vi "Teleop.vi"(10 "Match Info":T1={"Autonomous Elapsed Seconds"=0.0, "TeleOp Elapsed Seconds"=0.0, "Disabled Elapsed Seconds"=0.0, "Visited Autonomous"=FALSE, "Visited TeleOp"=FALSE, "Visited Disabled"=FALSE, "Autonomous Settings"={"Autonomous Style"=enum."Independent", "VI Refnum"=refnum}}, 11 "Call Context":T2) -> ()   [LabVIEW 2013]
doc: "This VI is called for each TeleOp packet received from the DS where the robot is not disabled. It is often used to read from the joysticks and update I/O or to update setpoints for timed control loops. It should complete and return within 20 milliseconds or it may miss DS packets."
uses:
  <vilib>/Rock Robotics/WPI/DriverStation/WPI_DriverStationDerivedRobotMode.ctl
  <vilib>/Rock Robotics/WPI/DriverStation/WPI_DriverStationMatch Info.ctl
  <vilib>/Rock Robotics/WPI/Solenoid/WPI_SolenoidValue.ctl
  Robot Global Data.vi
  <vilib>/Rock Robotics/WPI/Solenoid/Deprecated/WPI_SolenoidGetBool.vi
  <vilib>/Rock Robotics/WPI/Solenoid/WPI_SolenoidSetEnum.vi
  POT.vi
  Voltage.vi
  <vilib>/Rock Robotics/WPI/Joystick/WPI_JoystickGetSetRefNum.vi
  <vilib>/Rock Robotics/WPI/RobotDrive/WPI_RobotDriveGetSetRefNum.vi
panel:
  out "Voltage":dbl
  out "POT Value":dbl
  out "Numeric 1":dbl(slide) scale=0.0..100.0
  out "Boolean 2":bool
  out "Boolean 1":bool
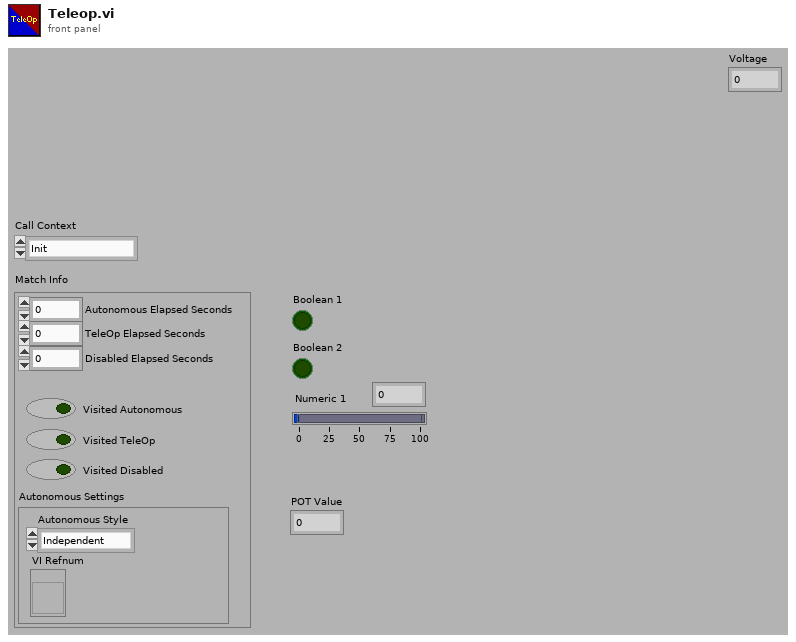
[diagram p1: front panel]
types:
  T1 = typedef "WPI_DriverStationMatch Info.ctl" = cluster{"Autonomous Elapsed Seconds":dbl, "TeleOp Elapsed Seconds":dbl, "Disabled Elapsed Seconds":dbl, "Visited Autonomous":bool, "Visited TeleOp":bool, "Visited Disabled":bool, "Autonomous Settings":cluster{"Autonomous Style":enum16{"Iterative", "Independent"}, "VI Refnum":refnum<vi>}}
  T2 = typedef "WPI_DriverStationDerivedRobotMode.ctl" = enum16{"Init", "Execute", "Stop"}
  T3 = typedef "WPI_JoystickDevRef.ctl" = cluster{"Device":T4}
  T4 = typedef "WPI_JoystickDeviceEnum.ctl" = enum16{"USB 1", "USB 2", "USB 3", "USB 4", "Kinect 1", "Kinect 2"}
  T5 = typedef "WPI_JoystickButtonState.ctl" = cluster{"Button 1":bool, "Button 2":bool, "Button 3":bool, "Button 4":bool, "Button 5":bool, "Button 6":bool, "Button 7":bool, "Button 8":bool, "Button 9":bool, "Button 10":bool, "Button 11":bool, "Button 12":bool}
  T6 = typedef "WPI_RobotDriveDevRef.ctl" = cluster{"DevStatus":errorcluster, "Motors[]":T7[], "Square Inputs":bool, "Max Output":dbl, "Isochronous":bool}
  T7 = typedef "WPI_MotorControlDeviceRef.ctl" = cluster{"DeviceStatus":errorcluster, "Type":enum16{"PWM", "CAN"}, "PWM":cluster{"Digital Module":T8, "PWM Channel":T9, "DeadBand":T10}, "CAN":cluster{"Device Number":u8, "Control Mode":T11, "Semaphore":T12, "Max Vout":dbl}, "Invert":bool, "TransformRef":T13, "InvTransformRef":T13}
  T8 = typedef "FPGA_TypedefDigitalModule.ctl" = enum16{"Digital Module 1", "Digital Module 2"}
  T9 = typedef "FPGA_DIOPWMChannel.ctl" = enum8{"PWM 1", "PWM 2", "PWM 3", "PWM 4", "PWM 5", "PWM 6", "PWM 7", "PWM 8", "PWM 9", "PWM 10", "Invalid"}
  T10 = typedef "WPI_PWMDeadband.ctl" = cluster{"Name":string, "maxPositivePwm":i32, "minPositivePwm":i32, "centerPwm":i32, "maxNegativePwm":i32, "minNegativePwm":i32, "angularRange":u16}
  T11 = typedef "WPI_CANJaguar_ControlMode.ctl" = enum8{"Percent VBus", "Current", "Speed", "Position", "Voltage"}
  T12 = typedef "Semaphore RefNum" = refnum<k1>
  T13 = typedef "WPI_PWMTransform_ConPane.ctl" = refnum<vi>
  T14 = cluster{"axis 1 (x)":dbl, "axis 2 (y)":dbl, "axis 3 (throttle)":dbl, "axis 4":dbl, "axis 5":dbl, "axis 6":dbl}
  T15 = typedef "WPI_SolenoidDevRef.ctl" = cluster{"DevStatus":errorcluster, "Solenoid Module":T16, "Forward Solenoid Channel":T17, "Reverse Solenoid Channel":T17}
  T16 = typedef "FPGA_TypedefSolenoidModule.ctl" = enum16{"Solenoid Module 1", "Solenoid Module 2"}
  T17 = typedef "WPI_SolenoidChannel.ctl" = enum8{"Solenoid 1", "Solenoid 2", "Solenoid 3", "Solenoid 4", "Solenoid 5", "Solenoid 6", "Solenoid 7", "Solenoid 8", "Invalid"}
  T18 = typedef "WPI_SolenoidValue.ctl" = enum16{"Off", "On", "Forward", "Reverse"}
  T19 = typedef "WPI_RelayDevRef.ctl" = cluster{"DevStatus":errorcluster, "Relay Channel":T20, "Digital Module":T8, "Relay Direction":T21}
  T20 = typedef "FPGA_DIORelayChannel.ctl" = enum8{"Relay 1", "Relay 2", "Relay 3", "Relay 4", "Relay 5", "Relay 6", "Relay 7", "Relay 8", "Invalid"}
  T21 = typedef "WPI_RelayDirection.ctl" = enum16{"Both directions", "Forward only", "Reverse only"}
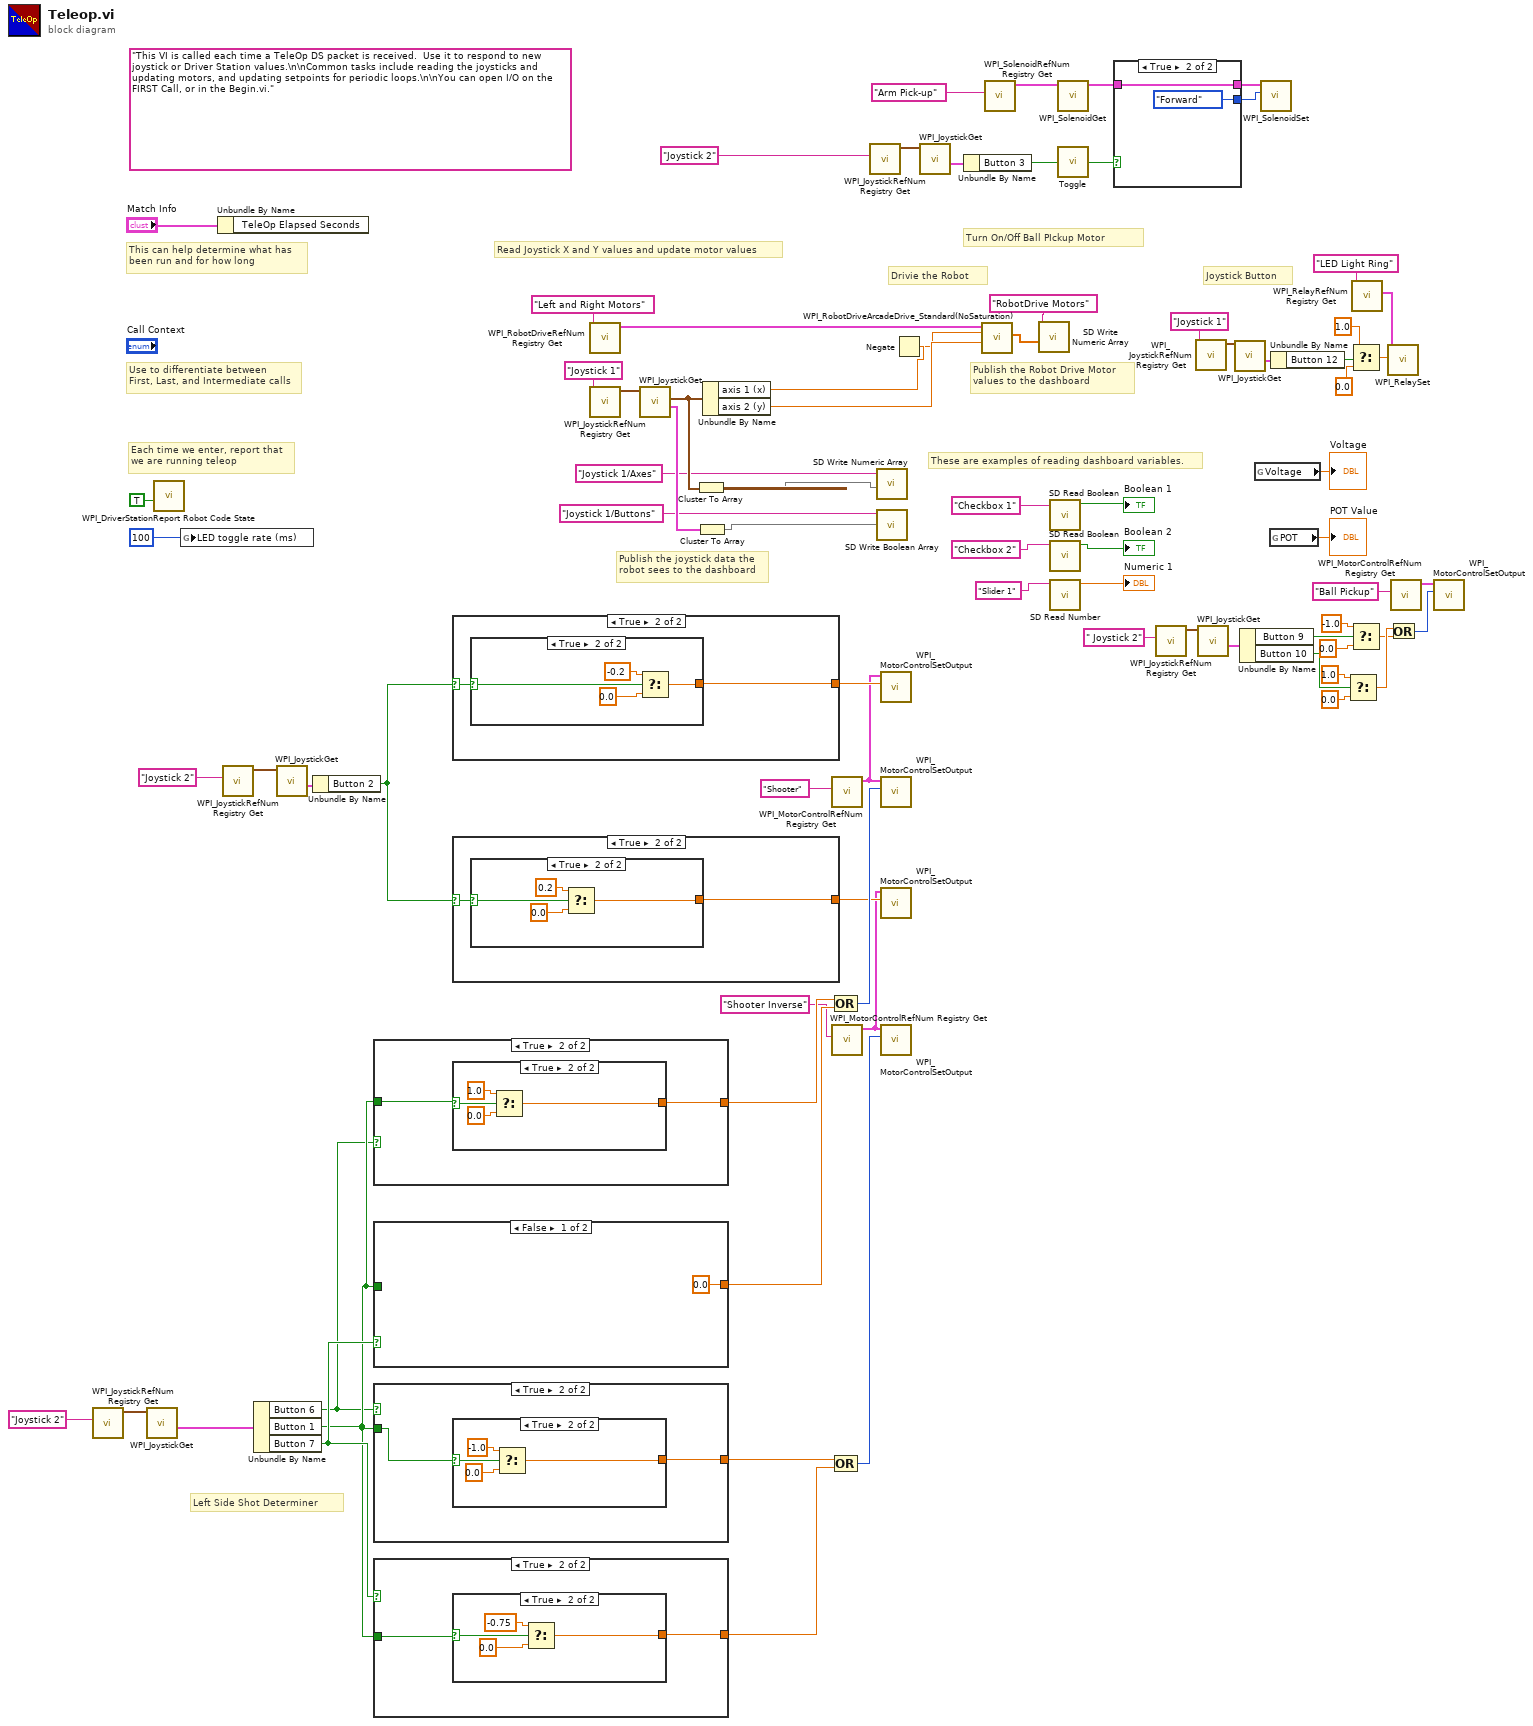
[diagram p0: block diagram]
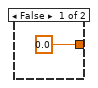
[diagram p2: hidden frame]
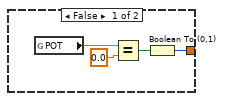
[diagram p3: hidden frame]
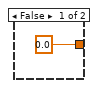
[diagram p4: hidden frame]
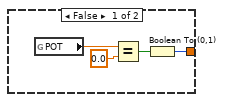
[diagram p5: hidden frame]
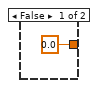
[diagram p6: hidden frame]
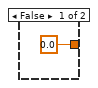
[diagram p7: hidden frame]
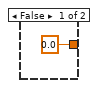
[diagram p8: hidden frame]
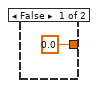
[diagram p9: hidden frame]
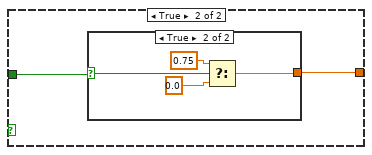
[diagram p10: hidden frame]
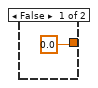
[diagram p11: hidden frame]
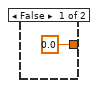
[diagram p12: hidden frame]
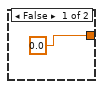
[diagram p13: hidden frame]
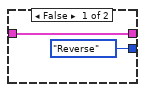
[diagram p14: hidden frame]
diagram:
  (unwired) "This VI is called each time a TeleOp DS packet is received.  Use it to respond to new joystick or Driver Station values.\n\nCommon tasks include reading the joysticks and updating motors, and updating setpoints for periodic loops.\n\nYou can open I/O on the FIRST Call, or in the Begin.vi."
  # "Left Side Shot Determiner"
  # "Turn On/Off Ball PIckup Motor"
  # "Joystick Button"
  # "Drivie the Robot"
  # "These are examples of reading dashboard variables."
  # "Publish the Robot Drive Motor\nvalues to the dashboard"
  # "Publish the joystick data the\nrobot sees to the dashboard"
  # "Each time we enter, report that\nwe are running teleop"
  # "Use to differentiate between\nFirst, Last, and Intermediate calls"
  # "This can help determine what has\nbeen run and for how long"
  # "Read Joystick X and Y values and update motor values"
  n1 = call <vilib>:"WPI_JoystickRefNum Registry Get.vi"("refnum name"="Joystick 2") -> ("JoystickDevRef"=w15:T3)  [unwired: 9 in, 1 out]
  n2 = call <vilib>:"WPI_JoystickGet.vi"("JoystickDevRef"=w15) -> ("Buttons"=w16:T5)  [unwired: 4 in, 2 out]
  n3 = call <vilib>:"WPI_DriverStationReport Robot Code State.vi"("TeleOp"=TRUE ("Autonomous")) -> ()  [unwired: 10 in, 1 out]
  n4 = global write "Robot Global Data.vi" "LED toggle rate (ms)"(u32 100 ("LED ms toggle rate")) -> ()
  n5 = Unbundle By Name("Match Info") -> ()  [unwired: 1 out]
  n6 = call <vilib>:"WPI_JoystickRefNum Registry Get.vi"("refnum name"="Joystick 2") -> ("JoystickDevRef"=w7:T3)  [unwired: 9 in, 1 out]
  n7 = Unbundle By Name(w16) -> ("Button 6"=w1:bool, "Button 1"=w2:bool, "Button 7"=w3:bool)
  n8 = call <vilib>:"WPI_JoystickGet.vi"("JoystickDevRef"=w7) -> ("Buttons"=w5:T5)  [unwired: 4 in, 2 out]
  n9 = Unbundle By Name(w5) -> ("Button 2"=w4:bool)
  n10 = case shown="True" w1 {
    tunnel: [0.0 ("f") w84] -> w20
    tunnel: w2 -> [_ w83]
    frame False {
    }
    frame True {
      n11 = case shown="True" w83 {
        selector: w83 -> [_ w87]
        tunnel: [0.0 ("y") w86] -> w84
        frame False {
        }
        frame True {
          n12 = Select(t=1.0, s=w87, f=0.0) -> (s? t:f=w86:dbl)
        }
      }
    }
  }
  n13 = case shown="False" w3 {
    tunnel: [0.0 ("f") w92] -> w21
    tunnel: w2 -> [_ w91]
    frame False {
    }
    frame True {
      n14 = case shown="True" w91 {
        selector: w91 -> [_ w95]
        tunnel: [0.0 ("y") w94] -> w92
        frame False {
        }
        frame True {
          n15 = Select(t=0.75, s=w95, f=0.0) -> (s? t:f=w94:dbl)
        }
      }
    }
  }
  n16 = case shown="True" w1 {
    tunnel: [0.0 ("f") w100] -> w17
    tunnel: w2 -> [_ w99]
    frame False {
    }
    frame True {
      n17 = case shown="True" w99 {
        selector: w99 -> [_ w103]
        tunnel: [0.0 ("y") w102] -> w100
        frame False {
        }
        frame True {
          n18 = Select(t=-1.0, s=w103, f=0.0) -> (s? t:f=w102:dbl)
        }
      }
    }
  }
  n19 = case shown="True" w3 {
    tunnel: [0.0 ("f") w108] -> w18
    tunnel: w2 -> [_ w107]
    frame False {
    }
    frame True {
      n20 = case shown="True" w107 {
        selector: w107 -> [_ w111]
        tunnel: [0.0 ("y") w110] -> w108
        frame False {
        }
        frame True {
          n21 = Select(t=-0.75, s=w111, f=0.0) -> (s? t:f=w110:dbl)
        }
      }
    }
  }
  n22 = case shown="True" w4 {
    selector: w4 -> [_ w115]
    tunnel: [0.0 ("f") w116] -> w10
    frame False {
    }
    frame True {
      n23 = case shown="True" w115 {
        selector: w115 -> [_ w122]
        tunnel: [w117 w121] -> w116
        frame False {
          n24 = global read "POT.vi" "POT"() -> (w119:dbl)
          n25 = Equal?(x=w119, y=0.0) -> (x = y?=w118:bool)
          n26 = Boolean To (0,1)(Boolean=w118) -> (0, 1=w117:i16)
        }
        frame True {
          n27 = Select(t=-0.2, s=w122, f=0.0) -> (s? t:f=w121:dbl)
        }
      }
    }
  }
  n28 = case shown="True" w4 {
    selector: w4 -> [_ w126]
    tunnel: [0.0 ("f") w127] -> w11
    frame False {
    }
    frame True {
      n29 = case shown="True" w126 {
        selector: w126 -> [_ w135]
        tunnel: [w128 w132] -> w127
        frame False {
          n30 = global read "POT.vi" "POT"() -> (w131:dbl)
          n31 = Equal?(x=w131, y=0.0) -> (x = y?=w129:bool)
          n32 = Boolean To (0,1)(Boolean=w129) -> (0, 1=w128:i16)
        }
        frame True {
          n33 = Select(t=0.2, s=w135, f=0.0) -> (s? t:f=w132:dbl)
        }
      }
    }
  }
  n34 = call <vilib>:"WPI_RobotDriveRefNum Registry Get.vi"("refnum name"="Left and Right Motors") -> ("RobotDriveDevRef"=w79:T6)  [unwired: 1 in, 9 out]
  n35 = call <vilib>:"WPI_JoystickRefNum Registry Get.vi"("refnum name"="Joystick 1") -> ("JoystickDevRef"=w76:T3)  [unwired: 1 in, 9 out]
  n36 = call <vilib>:"WPI_JoystickGet.vi"("JoystickDevRef"=w76) -> ("Buttons"=w73:T5, "Axes"=w70:T14)  [unwired: 1 in, 4 out]
  n37 = Cluster To Array(cluster=w70) -> (array=w69:dbl[])
  n38 = Cluster To Array(cluster=w73) -> (array=w72:bool[])
  n39 = Unbundle By Name(w70) -> ("axis 1 (x)"=w44:dbl, "axis 2 (y)"=w78:dbl)
  n40 = call <vilib>:"WPI_MotorControlRefNum Registry Get.vi"("refnum name"="Shooter") -> ("MotorControlDevRef"=w9:T7)  [unwired: 9 in, 1 out]
  n41 = call <vilib>:"WPI_MotorControlRefNum Registry Get.vi"("refnum name"="Shooter Inverse") -> ("MotorControlDevRef"=w8:T7)  [unwired: 9 in, 1 out]
  n42 = Compound Arithmetic op=OR(w20, w21) -> (w22:i32)
  n43 = Compound Arithmetic op=OR(w17, w18) -> (w19:i32)
  n44 = call <vilib>:"WPI_JoystickRefNum Registry Get.vi"("refnum name"="Joystick 2") -> ("JoystickDevRef"=w46:T3)  [unwired: 9 in, 1 out]
  n45 = call <vilib>:"SD Write Numeric Array.vi"("Numeric Array"=w69, "Name"="Joystick 1/Axes") -> ()  [unwired: 8 in, 2 out]
  n46 = call <vilib>:"SD Write Boolean Array.vi"("Boolean Array"=w72, "Name"="Joystick 1/Buttons") -> ()  [unwired: 8 in, 2 out]
  n47 = call <vilib>:"WPI_MotorControlSetOutput.vi"("Output"=w10, "MotorControlDevRef"=w9) -> ()  [unwired: 7 in, 3 out]
  n48 = call <vilib>:"WPI_MotorControlSetOutput.vi"("Output"=w22, "MotorControlDevRef"=w9) -> ()  [unwired: 7 in, 3 out]
  n49 = call <vilib>:"WPI_MotorControlSetOutput.vi"("Output"=w11, "MotorControlDevRef"=w8) -> ()  [unwired: 7 in, 3 out]
  n50 = call <vilib>:"WPI_MotorControlSetOutput.vi"("Output"=w19, "MotorControlDevRef"=w8) -> ()  [unwired: 7 in, 3 out]
  n51 = Negate(x=w44) -> (-x=w43:dbl)
  n52 = call <vilib>:"WPI_JoystickGet.vi"("JoystickDevRef"=w46) -> ("Buttons"=w45:T5)  [unwired: 4 in, 2 out]
  n53 = Unbundle By Name(w45) -> ("Button 3"=w42:bool)
  n54 = call <vilib>:"WPI_RobotDriveArcadeDrive_Standard(NoSaturation).vi"("Y axis value"=w78, "X axis value"=w43, "RobotDriveDevRef"=w79) -> ("Motor Values"=w66:dbl[])  [unwired: 1 in, 7 out]
  n55 = call <vilib>:"WPI_SolenoidRefNum Registry Get.vi"("refnum name"="Arm Pick-up") -> ("SolenoidDevRef"=w29:T15)  [unwired: 9 in, 1 out]
  n56 = call <vilib>:"SD Write Numeric Array.vi"("Numeric Array"=w66, "Name"="RobotDrive Motors") -> ()  [unwired: 8 in, 2 out]
  n57 = call <vilib>:"SD Read Boolean.vi"("Name"="Checkbox 1" ("refnum name")) -> ("Boolean"=→"Boolean 1":bool)  [unwired: 8 in, 2 out]
  n58 = call <vilib>:"SD Read Boolean.vi"("Name"="Checkbox 2" ("refnum name")) -> ("Boolean"=→"Boolean 2":bool)  [unwired: 8 in, 2 out]
  n59 = call <vilib>:"SD Read Number.vi"("Name"="Slider 1" ("refnum name")) -> ("Numeric"=→"Numeric 1":dbl)  [unwired: 8 in, 2 out]
  n60 = call-poly <vilib>:"WPI_SolenoidGet.vi"("SolenoidDevRef"=w29) -> ("SolenoidDevRef"=w27:T15)  [unwired: 8 in, 2 out]
  n61 = call "Toggle.vi"("Input"=w42) -> ("Toggled Output"=w28:bool)
  n62 = case shown="True" w28 {
    tunnel: w27 -> [w137 w139]
    tunnel: [w137 w139] -> w26
    tunnel: [WPI_SolenoidValue."Reverse" ("Value") WPI_SolenoidValue."Forward" ("Value")] -> w25
    frame False {
    }
    frame True {
    }
  }
  n63 = call <vilib>:"WPI_JoystickRefNum Registry Get.vi"("refnum name"=" Joystick 2") -> ("JoystickDevRef"=w35:T3)  [unwired: 9 in, 1 out]
  n64 = call <vilib>:"WPI_JoystickRefNum Registry Get.vi"("refnum name"="Joystick 1") -> ("JoystickDevRef"=w55:T3)  [unwired: 9 in, 1 out]
  n65 = call <vilib>:"WPI_JoystickGet.vi"("JoystickDevRef"=w35) -> ("Buttons"=w36:T5)  [unwired: 4 in, 2 out]
  n66 = call <vilib>:"WPI_JoystickGet.vi"("JoystickDevRef"=w55) -> ("Buttons"=w54:T5)  [unwired: 4 in, 2 out]
  n67 = Unbundle By Name(w36) -> ("Button 9"=w37:bool, "Button 10"=w33:bool)
  n68 = global read "Voltage.vi" "Voltage"() -> (→"Voltage":dbl)
  n69 = call-poly <vilib>:"WPI_SolenoidSet.vi"("Value"=w25, "SolenoidDevRef"=w26) -> ()  [unwired: 8 in, 2 out]
  n70 = global read "POT.vi" "POT"() -> (→"POT Value":dbl)
  n71 = Unbundle By Name(w54) -> ("Button 12"=w53:bool)
  n72 = Select(t=1.0, s=w33, f=0.0) -> (s? t:f=w32:dbl)
  n73 = Select(t=1.0, s=w53, f=0.0) -> (s? t:f=w52:dbl)
  n74 = Select(t=-1.0, s=w37, f=0.0) -> (s? t:f=w31:dbl)
  n75 = call <vilib>:"WPI_RelayRefNum Registry Get.vi"("refnum name"="LED Light Ring") -> ("RelayDevRef"=w59:T19)  [unwired: 9 in, 1 out]
  n76 = call <vilib>:"WPI_RelaySet.vi"("RelayValue"=w52, "RelayDevRef"=w59) -> ()  [unwired: 8 in, 2 out]
  n77 = Or(x=w32, y=w31) -> (x .or. y?=w30:i32)
  n78 = call <vilib>:"WPI_MotorControlRefNum Registry Get.vi"("refnum name"="Ball Pickup") -> ("MotorControlDevRef"=w49:T7)  [unwired: 9 in, 1 out]
  n79 = call <vilib>:"WPI_MotorControlSetOutput.vi"("Output"=w30, "MotorControlDevRef"=w49) -> ()  [unwired: 7 in, 3 out]
